vi "2013_04_30 Durability8 Main.vi"() -> ()   [LabVIEW 2013]
uses:
  MotorTypeDef.ctl
  <vilib>/DAQmx/write.llb/DAQmx Write (Counter Time 1Chan 1Samp).vi
  <vilib>/DAQmx/read.llb/DAQmx Read (Analog 1D Wfm NChan NSamp).vi
  <vilib>/Utility/TradDaqScaling.llb/Convert Thermistor Reading (waveform).vi
  <vilib>/DAQmx/miscellaneous.llb/DAQmx Fill In Error Info.vi
  <resource>/objmgr/daqmx.rc
panel:
  out "TotalSampPerChanAcquired":dbl
  out "AvailSampPerChan":u32
  in  "Y axis":u16(ring)=3 items=["RMS Current (A) 1"=1, "RMS Voltage (V) 1"=2, "RPM"=3, "Supply (V)"=4, "Torque (mNm)"=5, "Electrical Power (W)"=6, "Mechanical Power(W)"=7, "Motor Efficiency (%)"=8, "Source Current (A)"=10, "Supply Power (W)"=11, "ESC Efficiency (%)"=12, "Elapsed Time (h)"=0]
  in  "X axis":u16(ring) items=["RMS Current (A) 1"=1, "RMS Voltage (V) 1"=2, "RPM"=3, "Supply (V)"=4, "Torque (mNm)"=5, "Electrical Power (W)"=6, "Mechanical Power(W)"=7, "Motor Efficiency (%)"=8, "Source Current (A)"=10, "Supply Power (W)"=11, "ESC Efficiency (%)"=12, "Elapsed Time (h)"=0]
  out "XY Graph 2":cluster{"Array":dbl[], "Array":dbl[]}[](graph)
  out "Single Motor 2":waveform(dbl)[](graph)
  in  "Waveform":bool
  in  "Motor":dbl=1.0 min=1.0 max=8.0 step=1.0
  out "XY Graph":cluster{"Array":dbl[], "Array":dbl[]}[](graph)
  out "error out":errorcluster
  in  "Motor 8":T1 {"Elec Power In (W)" format="%.3g"; "Efficiency" format="%#_3g%%"; "Mech Pwr Out (W)" format="%.3g"; "Torque (mNm)" format="%.3g"; "Elapsed Time (h)" format="%.1f"; "Supply (V)" format="%.2f"; "RPM" scale=0.0..40000.0 scale format="%#_4p"}
  in  "Motor 7":T1={"Enabled"=FALSE, "Fail"=FALSE, "RPM"=0.0, "Motor"=enum."", "ESC"=enum."Phoenix", "Supply (V)"=0.0, "Test ID and Serial #"="test", "Comments"="", "Elapsed Time (h)"=0.0, "Counter"=0.0, "Torque (mNm)"=0.0, "Mech Pwr Out (W)"=0.0, "Efficiency"=0.0, "Elec Power In (W)"=0.0} {"Elec Power In (W)" format="%.3g"; "Efficiency" format="%#_3g%%"; "Mech Pwr Out (W)" format="%.3g"; "Torque (mNm)" format="%.3g"; "Elapsed Time (h)" format="%.1f"; "Supply (V)" format="%.2f"; "RPM" scale=0.0..40000.0 scale format="%#_4p"}
  in  "Motor 6":T1={"Enabled"=FALSE, "Fail"=FALSE, "RPM"=0.0, "Motor"=enum."", "ESC"=enum."Phoenix", "Supply (V)"=0.0, "Test ID and Serial #"="test", "Comments"="", "Elapsed Time (h)"=0.0, "Counter"=0.0, "Torque (mNm)"=0.0, "Mech Pwr Out (W)"=0.0, "Efficiency"=0.0, "Elec Power In (W)"=0.0} {"Elec Power In (W)" format="%.3g"; "Efficiency" format="%#_3g%%"; "Mech Pwr Out (W)" format="%.3g"; "Torque (mNm)" format="%.3g"; "Elapsed Time (h)" format="%.1f"; "Supply (V)" format="%.2f"; "RPM" scale=0.0..40000.0 scale format="%#_4p"}
  in  "Motor 5":T1={"Enabled"=FALSE, "Fail"=FALSE, "RPM"=0.0, "Motor"=enum."", "ESC"=enum."Phoenix", "Supply (V)"=0.0, "Test ID and Serial #"="test", "Comments"="", "Elapsed Time (h)"=0.0, "Counter"=0.0, "Torque (mNm)"=0.0, "Mech Pwr Out (W)"=0.0, "Efficiency"=0.0, "Elec Power In (W)"=0.0} {"Elec Power In (W)" format="%.3g"; "Efficiency" format="%#_3g%%"; "Mech Pwr Out (W)" format="%.3g"; "Torque (mNm)" format="%.3g"; "Elapsed Time (h)" format="%.1f"; "Supply (V)" format="%.2f"; "RPM" scale=0.0..40000.0 scale format="%#_4p"}
  in  "Motor 4":T1={"Enabled"=FALSE, "Fail"=FALSE, "RPM"=0.0, "Motor"=enum."", "ESC"=enum."Phoenix", "Supply (V)"=0.0, "Test ID and Serial #"="test", "Comments"="", "Elapsed Time (h)"=0.0, "Counter"=0.0, "Torque (mNm)"=0.0, "Mech Pwr Out (W)"=0.0, "Efficiency"=0.0, "Elec Power In (W)"=0.0} {"Elec Power In (W)" format="%.3g"; "Efficiency" format="%#_3g%%"; "Mech Pwr Out (W)" format="%.3g"; "Torque (mNm)" format="%.3g"; "Elapsed Time (h)" format="%.1f"; "Supply (V)" format="%.2f"; "RPM" scale=0.0..40000.0 scale format="%#_4p"}
  in  "Motor 3":T1={"Enabled"=FALSE, "Fail"=FALSE, "RPM"=0.0, "Motor"=enum."", "ESC"=enum."Phoenix", "Supply (V)"=0.0, "Test ID and Serial #"="test", "Comments"="", "Elapsed Time (h)"=0.0, "Counter"=0.0, "Torque (mNm)"=0.0, "Mech Pwr Out (W)"=0.0, "Efficiency"=0.0, "Elec Power In (W)"=0.0} {"Elec Power In (W)" format="%.3g"; "Efficiency" format="%#_3g%%"; "Mech Pwr Out (W)" format="%.3g"; "Torque (mNm)" format="%.3g"; "Elapsed Time (h)" format="%.1f"; "Supply (V)" format="%.2f"; "RPM" scale=0.0..40000.0 scale format="%#_4p"}
  in  "Motor 2":T1={"Enabled"=FALSE, "Fail"=FALSE, "RPM"=0.0, "Motor"=enum."", "ESC"=enum."Phoenix", "Supply (V)"=0.0, "Test ID and Serial #"="test", "Comments"="", "Elapsed Time (h)"=0.0, "Counter"=0.0, "Torque (mNm)"=0.0, "Mech Pwr Out (W)"=0.0, "Efficiency"=0.0, "Elec Power In (W)"=0.0} {"Elec Power In (W)" format="%.3g"; "Efficiency" format="%#_3g%%"; "Mech Pwr Out (W)" format="%.3g"; "Torque (mNm)" format="%.3g"; "Elapsed Time (h)" format="%.1f"; "Supply (V)" format="%.2f"; "RPM" scale=0.0..40000.0 scale format="%#_4p"}
  in  "Motor 1":T1={"Enabled"=FALSE, "Fail"=FALSE, "RPM"=0.0, "Motor"=enum."", "ESC"=enum."Phoenix", "Supply (V)"=0.0, "Test ID and Serial #"="test", "Comments"="", "Elapsed Time (h)"=0.0, "Counter"=0.0, "Torque (mNm)"=0.0, "Mech Pwr Out (W)"=0.0, "Efficiency"=0.0, "Elec Power In (W)"=0.0} {"Elec Power In (W)" format="%.3g"; "Efficiency" format="%#_3g%%"; "Mech Pwr Out (W)" format="%.3g"; "Torque (mNm)" format="%.3g"; "Elapsed Time (h)" format="%.1f"; "Supply (V)" format="%.2f"; "RPM" scale=0.0..40000.0 scale format="%#_4p"}
  out "Motor Temp":dbl(slide) scale=65.0..110.0
  out "Tank Temp":dbl(slide) scale=65.0..110.0
  in  "Temp Probe\nOn Motor":dbl=9.0
  out "loop time (ms)":u32
  in  "stop":bool
  in  "Unlock PWM":bool=TRUE
  in  "PWM 2":dbl(slide)=100.0 min=0.0 max=100.0 step=5.0 scale=0.0..100.0
  in  "PWM 1":dbl(slide) min=0.0 max=100.0 step=5.0 scale=0.0..100.0
  # "Enable"
  # "Fail"
  # "Enable"
  # "Fail"
  # "Enable"
  # "Fail"
  # "Enable"
  # "Fail"
  # "Enable"
  # "Fail"
  # "Enable"
  # "Fail"
  # "Enable"
  # "Fail"
  # "Enable"
  # "Fail"
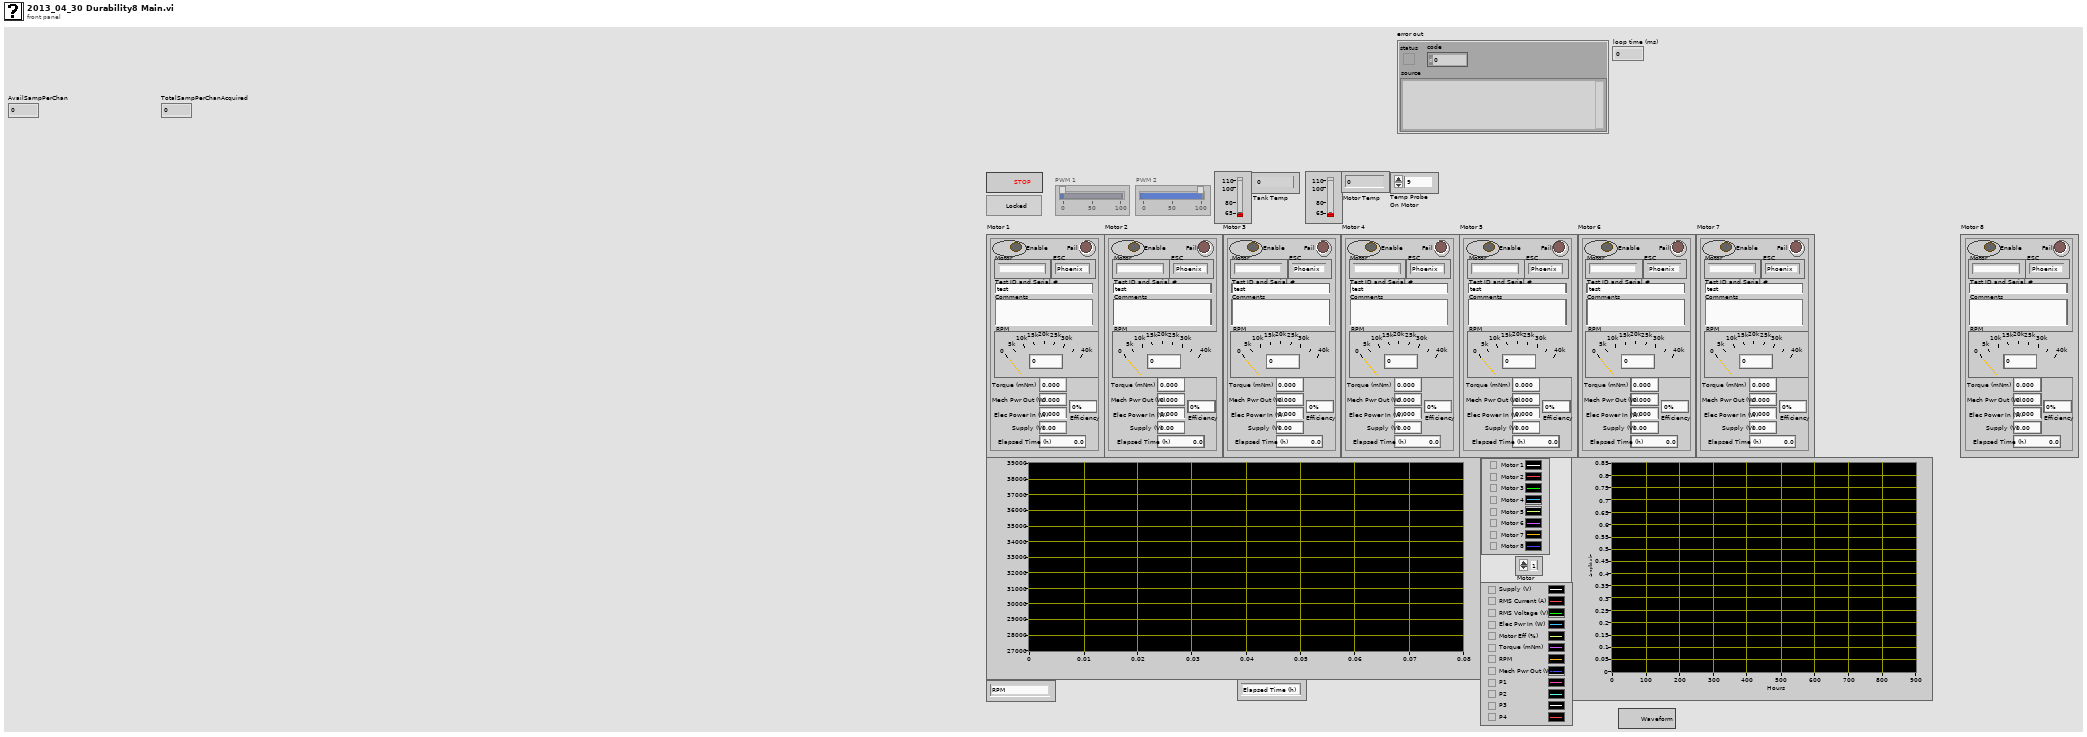
[diagram p1: front panel]
types:
  T1 = typedef "MotorTypeDef.ctl" = cluster{"Enabled":bool, "Fail":bool, "RPM":dbl, "Motor":enum16{"", "Maxon EC6 6V", "Maxon EC4 6V", "FH 0620 6V", "FH 0620 12V"}, "ESC":enum16{"Phoenix", "Maxon", "FH 1801"}, "Supply (V)":dbl, "Test ID and Serial #":string, "Comments":string, "Elapsed Time (h)":dbl, "Counter":dbl, "Torque (mNm)":dbl, "Mech Pwr Out (W)":dbl, "Efficiency":dbl, "Elec Power In (W)":dbl}
  T2 = enum8{"Enabled", "Disabled", "Disabled and Grayed Out"}
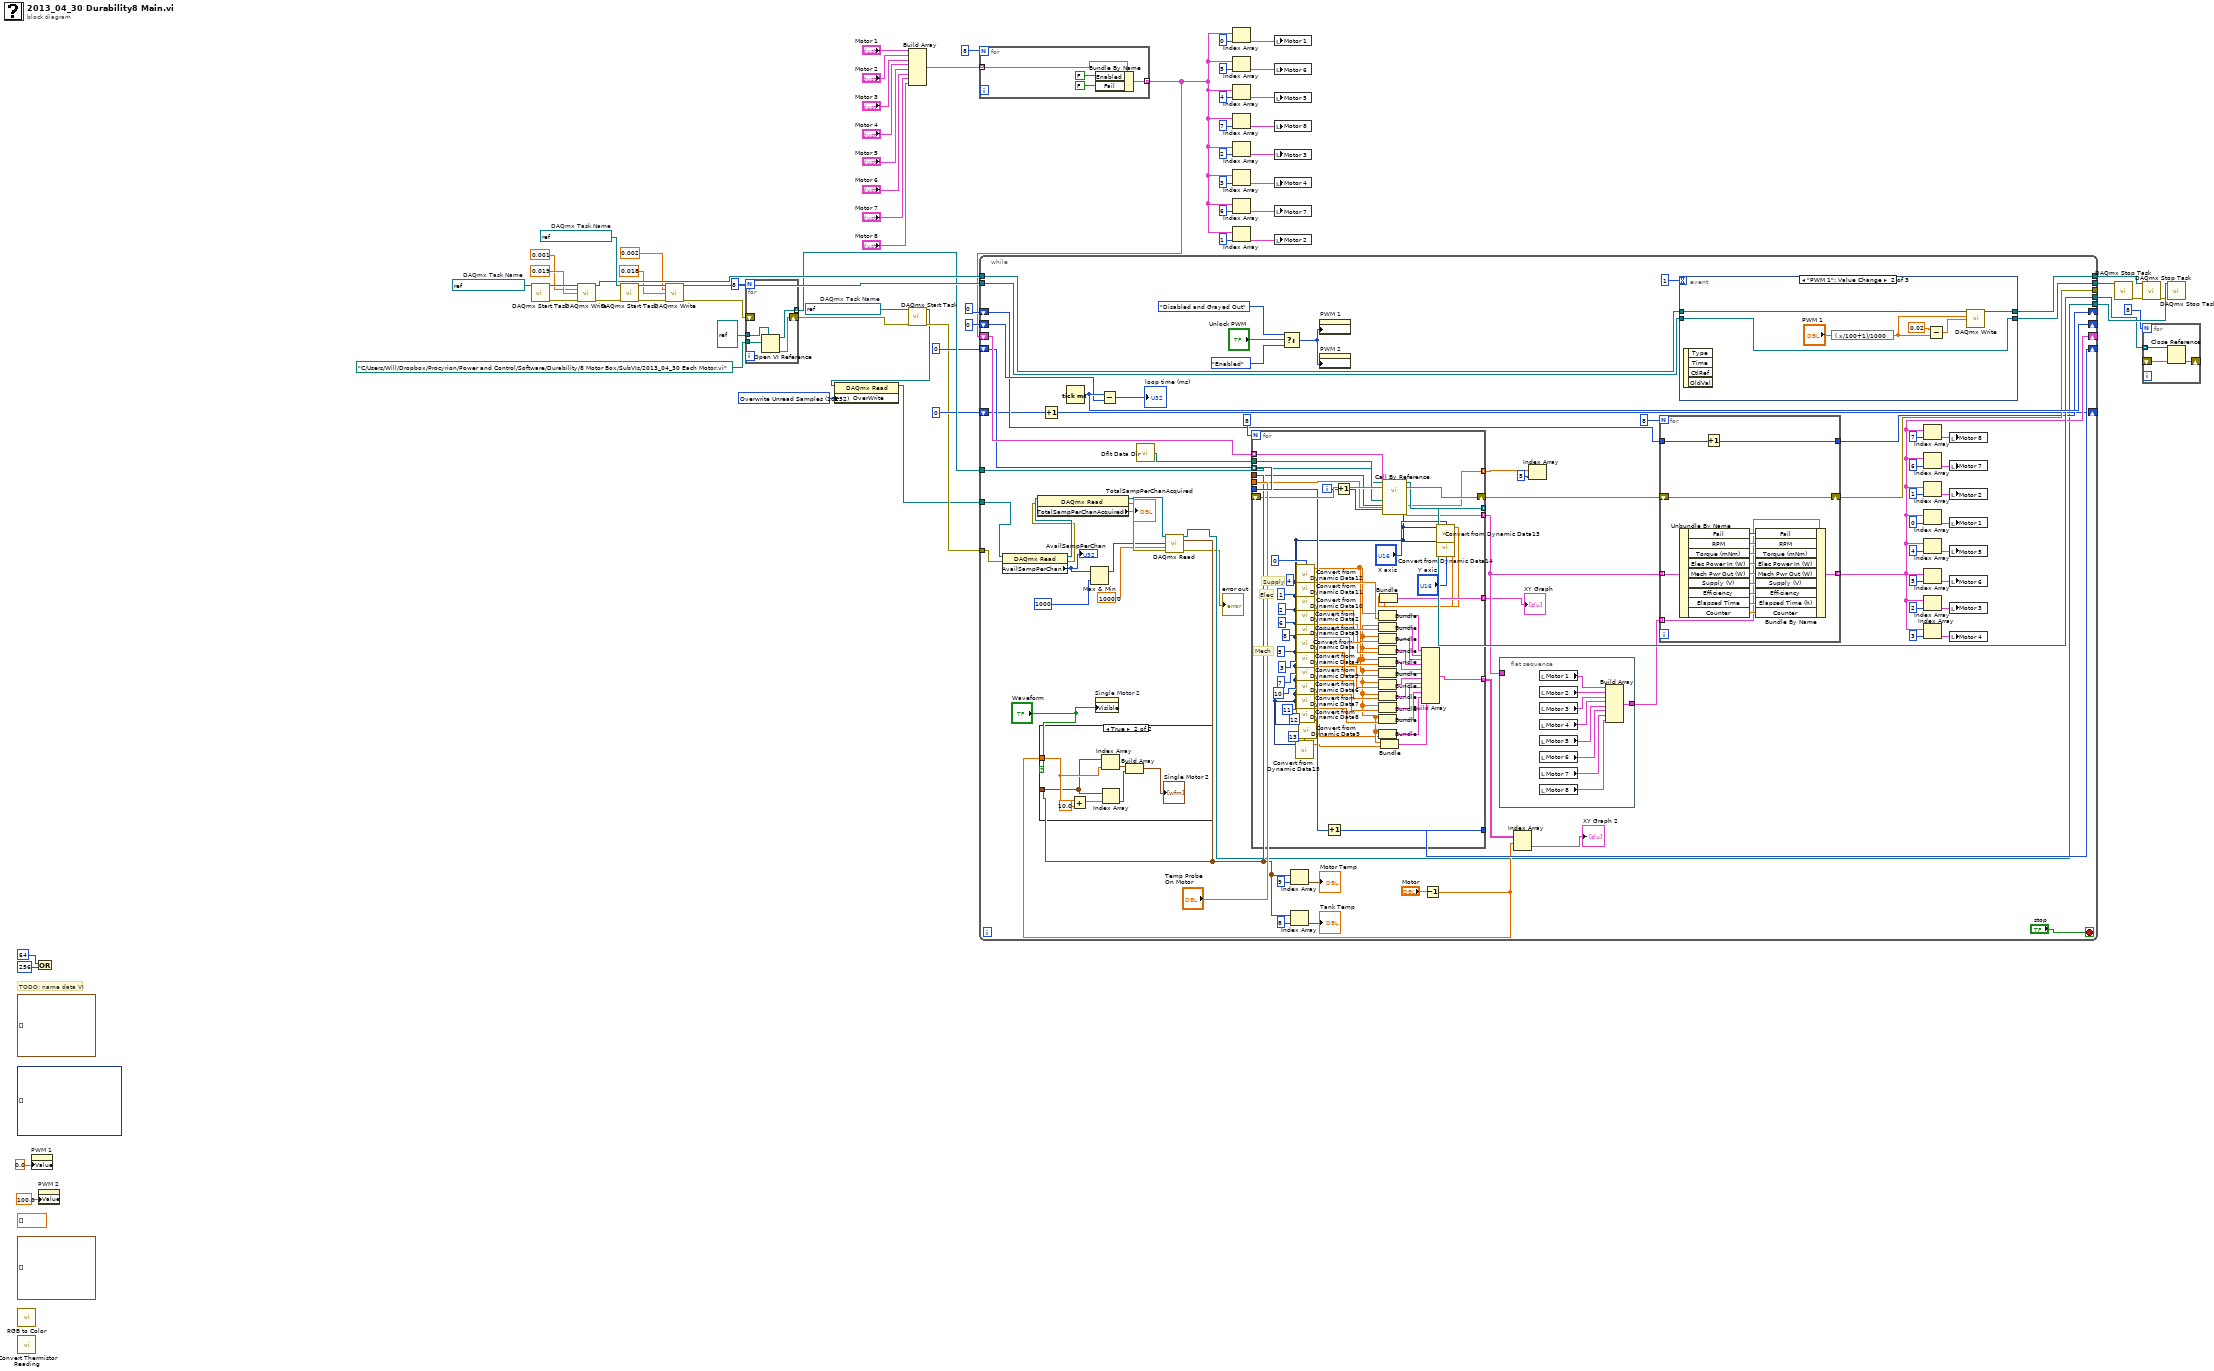
[diagram p0: block diagram]
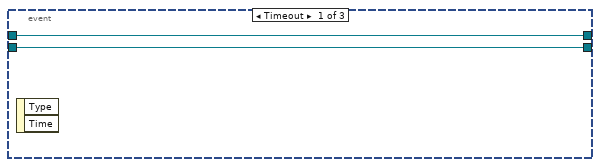
[diagram p3: hidden frame]
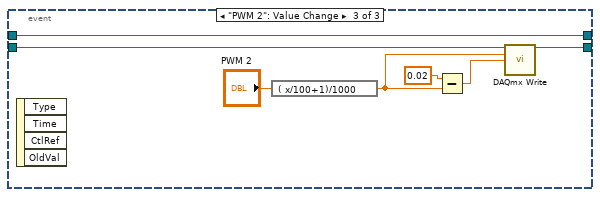
[diagram p4: hidden frame]
diagram:
  w1 = 10252 items=["Overwrite Unread Samples"=10252, "Do Not Overwrite Unread Samples"=10159] ("OverWrite")
  (unwired) dynamicdata[] []
  (unwired) dbl[] [] ("History Data")
  (unwired) waveform(dbl)[][] [] ("History Data")
  (unwired) waveform(dbl)[][] [] ("History Data")
  w63 = refnum<k21> "Durability8 PWM2"  # DAQmx Task Name
  w64 = refnum<k21> "Durability8 PWM1"  # DAQmx Task Name
  w66 = refnum<k21> "Durability8 Acquire"  # DAQmx Task Name
  # "TODO: name data VI"
  n1 = call <vilib>:"RGB to Color.vi"() -> ()  [unwired: 3 in, 1 out]
  n2 = call-poly <vilib>:"Convert Thermistor Reading.vi"() -> ()  [unwired: 7 in, 1 out]
  n3 = property on="PWM 1" class="Slide (strict)"("Value"=0.0 ("PWM 1")) -> ()  [unwired: 2 in, 2 out]
  n4 = Compound Arithmetic op=OR(64 ("options"), 256 ("options")) -> ()  [unwired: 1 out]
  n5 = property on="PWM 2" class="Slide (strict)"("Value"=100.0 ("PWM 2")) -> ()  [unwired: 2 in, 2 out]
  n6 = call <vilib>:"DAQmx Start Task.vi"("task/channels in"=w64) -> ("task out"=w60:refnum<k21>, "error out"=w58:errorcluster)  [unwired: 13 in]
  n7 = call-poly <vilib>:"DAQmx Write.vi"("task/channels in"=w60, "high time"=0.001 ("data"), "low time"=0.019 ("data"), "error in"=w58) -> ("task out"=w62:refnum<k21>, "error out"=w57:errorcluster)  [unwired: 9 in, 1 out]
  n8 = call <vilib>:"DAQmx Start Task.vi"("task/channels in"=w63, "error in"=w57) -> ("task out"=w59:refnum<k21>, "error out"=w56:errorcluster)  [unwired: 12 in]
  n9 = call-poly <vilib>:"DAQmx Write.vi"("task/channels in"=w59, "high time"=0.002 ("data"), "low time"=0.018 ("data"), "error in"=w56) -> ("task out"=w61:refnum<k21>, "error out"=w25:errorcluster)  [unwired: 9 in, 1 out]
  n10 = for {
    N: 8 -> [_]
    tunnel: path "C:/Users/Will/Dropbox/Procyrion/Power and Control/Software/Durability/8 Motor Box/SubVIs/2013_04_30 Each Motor.vi" -> [w70]
    tunnel: [w69] -> w41 mode=indexing
    tunnel: refnum<vi> refnum ("type specifier VI Refnum (for type only)") -> [w68]
    shift-right: [w67] -> w26
    shift-left: w25 -> [_]
    n11 = Open VI Reference(type specifier VI Refnum (for type only)=w68, vi path=w70) -> (vi reference=w69:refnum<vi>, error out=w67:errorcluster)  [unwired: 4 in]
  }
  n12 = Build Array("Motor 1", "Motor 2", "Motor 3", "Motor 4", "Motor 5", "Motor 6", "Motor 7", "Motor 8") -> (w22:T1[])
  n13 = call <vilib>:"DAQmx Start Task.vi"("task/channels in"=w66, "error in"=w26) -> ("task out"=w3:refnum<k21>, "error out"=w24:errorcluster)  [unwired: 12 in]
  n14 = property class="DAQmx Read"(reference=w3, "OverWrite"=w1) -> (reference out=w2:refnum<k21>)  [unwired: 1 in, 1 out]
  n15 = for {
    N: 8 -> [_]
    tunnel: w22 -> [w74] mode=indexing
    tunnel: [w71] -> w5 mode=indexing
    n16 = Bundle By Name(cluster=w74, "Enabled"=FALSE, "Fail"=FALSE) -> (w71:T1)
  }
  n17 = while {
    tunnel: w2 -> [w89]
    tunnel: [w93] -> w65
    tunnel: w24 -> [w88]
    shift-right: [w143] -> _
    shift-left: u32 0 ("millisecond timer value") -> [w142]
    tunnel: w62 -> [w135]
    tunnel: w61 -> [w76]
    tunnel: [w134] -> w55
    tunnel: [w133] -> w48
    tunnel: w41 -> [w130]
    tunnel: [w129] -> w37
    shift-right: [w111] -> _
    shift-left: w5 -> [w110]
    tunnel: [w109] -> _
    shift-right: [w106] -> _
    shift-left: 0 ("for") -> [w107]
    shift-right: [w104] -> _
    shift-left: 0 ("for") -> [w105]
    shift-right: [w102] -> _
    shift-left: 0 ("for") -> [w103]
    stop <- "stop" stop-if-true
    n18 = property class="DAQmx Read"(reference=w89, error in=w88) -> (reference out=w87:refnum<k21>, error out=w86:errorcluster, "AvailSampPerChan"=w85:u32)
    "AvailSampPerChan" <- w85
    n19 = property class="DAQmx Read"(reference=w87, error in=w86) -> (reference out=w83:refnum<k21>, error out=w82:errorcluster, "TotalSampPerChanAcquired"=→"TotalSampPerChanAcquired":dbl)
    n20 = Increment(x=w103) -> (x+1=w102:i32)
    n21 = Tick Count (ms)() -> (millisecond timer value=w143:u32)
    n22 = Max & Min(x=w85, y=1000 ("number of samples per channel")) -> (max(x,y)=w80:u32)  [unwired: 1 out]
    n23 = property on="Single Motor 2" class="WFGraph (strict)"("Visible"="Waveform") -> ()  [unwired: 2 in, 2 out]
    n24 = Subtract(x=w143, y=w142) -> (x-y=→"loop time (ms)":u32)
    n25 = call <vilib>:"Dflt Data Dir.vi"() -> ("App:Default Data Directory"=w75:path)
    n26 = call-poly <vilib>:"DAQmx Read.vi"("task/channels in"=w83, "number of samples per channel"=w80, "timeout"=1000.0, "error in"=w82) -> ("task out"=w93:refnum<k21>, "data"=w96:waveform(dbl)[], "error out"=→"error out":errorcluster)  [unwired: 9 in]
    n27 = for {
      N: 8 -> [_]
      tunnel: w96 -> [w249]
      tunnel: w75 -> [w250]
      tunnel: w130 -> [w216] mode=indexing
      shift-right: [w253] -> w108
      shift-left: _ -> [w252]
      tunnel: [w247] -> w129 mode=indexing
      tunnel: [w246] -> w100 mode=indexing
      tunnel: w110 -> [w204] mode=indexing
      tunnel: w107 -> [w245]
      tunnel: [w244] -> w106
      tunnel: "Temp Probe\nOn Motor" -> [w243]
      tunnel: [w242] -> w98 mode=indexing
      tunnel: [w231] -> w92 mode=indexing
      tunnel: [w203] -> w78 mode=indexing
      i -> [w251]
      # "Mech"
      # "Elec"
      # "Supply"
      n28 = Increment(x=w245) -> (x+1=w244:i32)
      n29 = Increment(x=w251) -> (x+1=w248:i32)
      n30 = call-by-ref "?"(reference=w216, error in=w252, "Temp On"=w243, "Motor #"=w248, "data"=w249, "File Path"=w250, "Motor Typedef"=w204) -> (reference out=w247:refnum<vi>, error out=w253:errorcluster, "Final Out"=w200:dynamicdata, "Counter"=w203:dbl, "Motor Typedef Out"=w246:T1)  [unwired: 4 in]
      n31 = call "Convert from Dynamic Data15"("Dynamic Data Type"=w200, "Channel"=13) -> ("Array"=w197:dbl[])  [unwired: 2 in]
      n32 = call "Convert from Dynamic Data12"("Dynamic Data Type"=w200, "Channel"=0) -> ("Array"=w199:dbl[])  [unwired: 2 in]
      n33 = call "Convert from Dynamic Data11"("Dynamic Data Type"=w200, "Channel"=4) -> ("Array"=w230:dbl[])  [unwired: 2 in]
      n34 = call "Convert from Dynamic Data10"("Dynamic Data Type"=w200, "Channel"=1) -> ("Array"=w229:dbl[])  [unwired: 2 in]
      n35 = call "Convert from Dynamic Data2"("Dynamic Data Type"=w200, "Channel"=2) -> ("Array"=w228:dbl[])  [unwired: 2 in]
      n36 = call "Convert from Dynamic Data3"("Dynamic Data Type"=w200, "Channel"=6) -> ("Array"=w227:dbl[])  [unwired: 2 in]
      n37 = call "Convert from Dynamic Data"("Dynamic Data Type"=w200, "Channel"=8) -> ("Array"=w226:dbl[])  [unwired: 2 in]
      n38 = call "Convert from Dynamic Data4"("Dynamic Data Type"=w200, "Channel"=5) -> ("Array"=w225:dbl[])  [unwired: 2 in]
      n39 = call "Convert from Dynamic Data5"("Dynamic Data Type"=w200, "Channel"=3) -> ("Array"=w224:dbl[])  [unwired: 2 in]
      n40 = call "Convert from Dynamic Data6"("Dynamic Data Type"=w200, "Channel"=7) -> ("Array"=w223:dbl[])  [unwired: 2 in]
      n41 = call "Convert from Dynamic Data7"("Dynamic Data Type"=w200, "Channel"=10) -> ("Array"=w222:dbl[])  [unwired: 2 in]
      n42 = call "Convert from Dynamic Data8"("Dynamic Data Type"=w200, "Channel"=11) -> ("Array"=w221:dbl[])  [unwired: 2 in]
      n43 = call "Convert from Dynamic Data9"("Dynamic Data Type"=w200, "Channel"=12) -> ("Array"=w198:dbl[])  [unwired: 2 in]
      n44 = Bundle("Array"=w199, "Array"=w230) -> (w232:cluster{"Array":dbl[], "Array":dbl[]})  [unwired: 1 in]
      n45 = Bundle("Array"=w199, "Array"=w229) -> (w233:cluster{"Array":dbl[], "Array":dbl[]})  [unwired: 1 in]
      n46 = Bundle("Array"=w199, "Array"=w228) -> (w234:cluster{"Array":dbl[], "Array":dbl[]})  [unwired: 1 in]
      n47 = Bundle("Array"=w199, "Array"=w227) -> (w235:cluster{"Array":dbl[], "Array":dbl[]})  [unwired: 1 in]
      n48 = Bundle("Array"=w199, "Array"=w226) -> (w236:cluster{"Array":dbl[], "Array":dbl[]})  [unwired: 1 in]
      n49 = Bundle("Array"=w199, "Array"=w225) -> (w237:cluster{"Array":dbl[], "Array":dbl[]})  [unwired: 1 in]
      n50 = Bundle("Array"=w199, "Array"=w224) -> (w238:cluster{"Array":dbl[], "Array":dbl[]})  [unwired: 1 in]
      n51 = Bundle("Array"=w199, "Array"=w223) -> (w239:cluster{"Array":dbl[], "Array":dbl[]})  [unwired: 1 in]
      n52 = Bundle("Array"=w199, "Array"=w222) -> (w241:cluster{"Array":dbl[], "Array":dbl[]})  [unwired: 1 in]
      n53 = Bundle("Array"=w199, "Array"=w221) -> (w240:cluster{"Array":dbl[], "Array":dbl[]})  [unwired: 1 in]
      n54 = Bundle("Array"=w199, "Array"=w198) -> (w196:cluster{"Array":dbl[], "Array":dbl[]})  [unwired: 1 in]
      n55 = Bundle("Array"=w199, "Array"=w197) -> (w195:cluster{"Array":dbl[], "Array":dbl[]})  [unwired: 1 in]
      n56 = Build Array(w232, w233, w234, w235, w236, w237, w238, w239, w241, w240, w196, w195) -> (w231:cluster{"Array":dbl[], "Array":dbl[]}[])
      n57 = call "Convert from Dynamic Data13"("Dynamic Data Type"=w200, "Channel"="X axis") -> ("Array"=w218:dbl[])  [unwired: 2 in]
      n58 = call "Convert from Dynamic Data14"("Dynamic Data Type"=w200, "Channel"="Y axis") -> ("Array"=w217:dbl[])  [unwired: 2 in]
      n59 = Bundle("Array"=w218, "Array"=w217) -> (w242:cluster{"Array":dbl[], "Array":dbl[]})  [unwired: 1 in]
    }
    "XY Graph" <- w98
    n60 = Select(t=T2."Disabled and Grayed Out" ("Disabled"), s="Unlock PWM", f=T2."Enabled" ("Disabled")) -> (s? t:f=w147:T2)
    n61 = Index Array(array=w96, index=9) -> (element=→"Motor Temp":waveform(dbl))
    n62 = Index Array(array=w96, index=8) -> (element=→"Tank Temp":waveform(dbl))
    n63 = property on="PWM 1" class="Slide (strict)"("DisabledEnum"=w147) -> ()  [unwired: 2 in, 2 out]
    n64 = property on="PWM 2" class="Slide (strict)"("DisabledEnum"=w147) -> ()  [unwired: 2 in, 2 out]
    n65 = Decrement(x="Motor") -> (x-1=w95:dbl)
    n66 = case shown="True" "Waveform" {
      tunnel: w96 -> [_ w152]
      tunnel: w95 -> [_ w153]
      frame False {
      }
      frame True {
        n67 = Add(x=w153, y=10.0) -> (x+y=w151:dbl)
        n68 = Index Array(array=w152, index=w153) -> (element=w150:waveform(dbl))
        n69 = Index Array(array=w152, index=w151) -> (element=w149:waveform(dbl))
        n70 = Build Array(w150, w149) -> (→"Single Motor 2":waveform(dbl)[])
      }
    }
    n71 = flat-sequence {
      tunnel: [w156] -> w101
      tunnel: w100 -> [_]
      frame #0 {
        n72 = local read "Motor 1"() -> (w157:T1)
        n73 = local read "Motor 2"() -> (w158:T1)
        n74 = local read "Motor 3"() -> (w159:T1)
        n75 = local read "Motor 4"() -> (w160:T1)
        n76 = local read "Motor 5"() -> (w161:T1)
        n77 = local read "Motor 6"() -> (w162:T1)
        n78 = local read "Motor 7"() -> (w163:T1)
        n79 = local read "Motor 8"() -> (w155:T1)
        n80 = Build Array(w157, w158, w159, w160, w161, w162, w163, w155) -> (w156:T1[])
      }
    }
    n81 = Index Array(array=w92, index (row)=w95) -> (element=→"XY Graph 2":cluster{"Array":dbl[], "Array":dbl[]}[])  [unwired: 1 in]
    n82 = Index Array(array=w78, index=5) -> ()  [unwired: 1 out]
    n83 = for {
      N: 8 -> [_]
      tunnel: w101 -> [w169] mode=indexing
      tunnel: [w168] -> w111 mode=indexing
      tunnel: w100 -> [w167] mode=indexing
      shift-right: [w166] -> w109
      shift-left: w108 -> [w166]
      tunnel: [w164] -> w104
      tunnel: w105 -> [w165]
      n84 = Unbundle By Name(w167) -> ("Fail"=w178:bool, "RPM"=w177:dbl, "Torque (mNm)"=w176:dbl, "Elec Power In (W)"=w175:dbl, "Mech Pwr Out (W)"=w174:dbl, "Supply (V)"=w173:dbl, "Efficiency"=w172:dbl, "Elapsed Time"=w171:dbl, "Counter"=w170:dbl)
      n85 = Increment(x=w165) -> (x+1=w164:i32)
      n86 = Bundle By Name(cluster=w169, "Fail"=w178, "RPM"=w177, "Torque (mNm)"=w176, "Elec Power In (W)"=w175, "Mech Pwr Out (W)"=w174, "Supply (V)"=w173, "Efficiency"=w172, "Elapsed Time (h)"=w171, "Counter"=w170) -> (w168:T1)
    }
    n87 = event shown="[1] \"PWM 1\": Value Change" {
      selector: _ -> [_ _ _]
      dyn-events: _ -> [_ _ _]
      timeout: 1 -> [_ _ _]
      tunnel: w135 -> [w180 w183 w189]
      tunnel: w76 -> [w179 w181 w188]
      tunnel: [w180 w182 w189] -> w134
      tunnel: [w179 w181 w190] -> w133
      event Timeout {
        n88 = event-data() -> ()  [unwired: 1 in, 2 out]
      }
      event "PWM 1": Value Change {
        n89 = event-data() -> ()  [unwired: 1 in, 4 out]
        n90 = expression code="( x/100+1)/1000"("PWM 1") -> (w184:dbl)
        n91 = Subtract(x=0.02 ("y"), y=w184) -> (x-y=w185:dbl)
        n92 = call-poly <vilib>:"DAQmx Write.vi"("task/channels in"=w183, "high time"=w184, "low time"=w185) -> ("task out"=w182:refnum<k21>)  [unwired: 10 in, 2 out]
      }
      event "PWM 2": Value Change {
        n93 = event-data() -> ()  [unwired: 1 in, 4 out]
        n94 = expression code="( x/100+1)/1000"("PWM 2") -> (w194:dbl)
        n95 = Subtract(x=0.02, y=w194) -> (x-y=w192:dbl)
        n96 = call-poly <vilib>:"DAQmx Write.vi"("task/channels in"=w188, "high time"=w194, "low time"=w192) -> ("task out"=w190:refnum<k21>)  [unwired: 10 in, 2 out]
      }
    }
    n97 = Index Array(array=w111, index=7) -> (element=w118:T1)
    n98 = Index Array(array=w111, index=6) -> (element=w117:T1)
    n99 = Index Array(array=w111, index=1) -> (element=w112:T1)
    n100 = Index Array(array=w111, index=0) -> (element=w127:T1)
    n101 = Index Array(array=w111, index=4) -> (element=w115:T1)
    n102 = Index Array(array=w111, index=5) -> (element=w116:T1)
    n103 = Index Array(array=w111, index=2) -> (element=w113:T1)
    n104 = Index Array(array=w111, index=3) -> (element=w114:T1)
    n105 = local write "Motor 8"(w118) -> ()
    n106 = local write "Motor 7"(w117) -> ()
    n107 = local write "Motor 2"(w112) -> ()
    n108 = local write "Motor 1"(w127) -> ()
    n109 = local write "Motor 5"(w115) -> ()
    n110 = local write "Motor 6"(w116) -> ()
    n111 = local write "Motor 3"(w113) -> ()
    n112 = local write "Motor 4"(w114) -> ()
  }
  n113 = Index Array(array=w5, index=0) -> (element=w21:T1)
  n114 = Index Array(array=w5, index=5) -> (element=w10:T1)
  n115 = Index Array(array=w5, index=4) -> (element=w9:T1)
  n116 = Index Array(array=w5, index=7) -> (element=w12:T1)
  n117 = Index Array(array=w5, index=2) -> (element=w7:T1)
  n118 = Index Array(array=w5, index=3) -> (element=w8:T1)
  n119 = Index Array(array=w5, index=6) -> (element=w11:T1)
  n120 = Index Array(array=w5, index=1) -> (element=w6:T1)
  n121 = local write "Motor 1"(w21) -> ()
  n122 = local write "Motor 6"(w10) -> ()
  n123 = local write "Motor 5"(w9) -> ()
  n124 = local write "Motor 8"(w12) -> ()
  n125 = local write "Motor 3"(w7) -> ()
  n126 = local write "Motor 4"(w8) -> ()
  n127 = local write "Motor 7"(w11) -> ()
  n128 = local write "Motor 2"(w6) -> ()
  n129 = call <vilib>:"DAQmx Stop Task.vi"("task/channels in"=w48) -> ("error out"=w54:errorcluster)  [unwired: 13 in, 1 out]
  n130 = call <vilib>:"DAQmx Stop Task.vi"("task/channels in"=w55, "error in"=w54) -> ("error out"=w53:errorcluster)  [unwired: 12 in, 1 out]
  n131 = for {
    N: 8 -> [_]
    shift-right: [w256] -> _
    shift-left: _ -> [w254]
    tunnel: w37 -> [w255] mode=indexing
    n132 = Close Reference(reference=w255, error in (no error)=w254) -> (error out=w256:errorcluster)
  }
  n133 = call <vilib>:"DAQmx Stop Task.vi"("task/channels in"=w65, "error in"=w53) -> ()  [unwired: 12 in, 2 out]
